vi "PID.vi"(0 "Refnum in":refnum<k21>, 1 "PID On/Off":bool, 2 "VISA resource name":refnum<visa-resource-name>, 3 "error in (no error)":errorcluster, 4 "Parameters":cluster{"P":dbl, "I":dbl, "D":dbl}, 5 "Plus Resistance":dbl, 6 "Goal Temperature (K)":dbl, 7 "Temperature":dbl) -> (8 "PID signal":dbl format="%.2f", 10 "error out":errorcluster)   [LabVIEW 2017]
uses:
  <vilib>/DAQmx/read.llb/DAQmx Read (Analog 1D DBL NChan 1Samp).vi
  <vilib>/DAQmx/miscellaneous.llb/DAQmx Fill In Error Info.vi
  <vilib>/addons/control/pid/pid.llb/PID (DBL).vi
  <vilib>/addons/control/pid/NI_PID_pid.lvlib
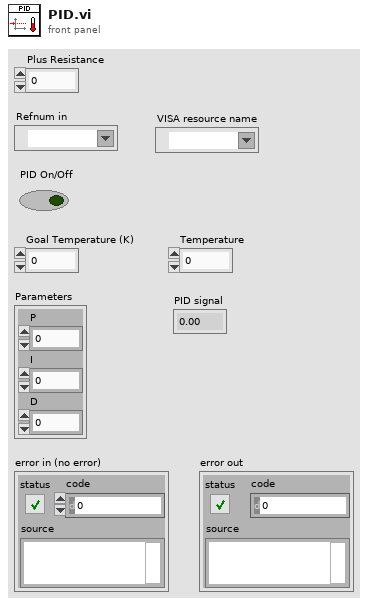
[diagram p1: front panel]
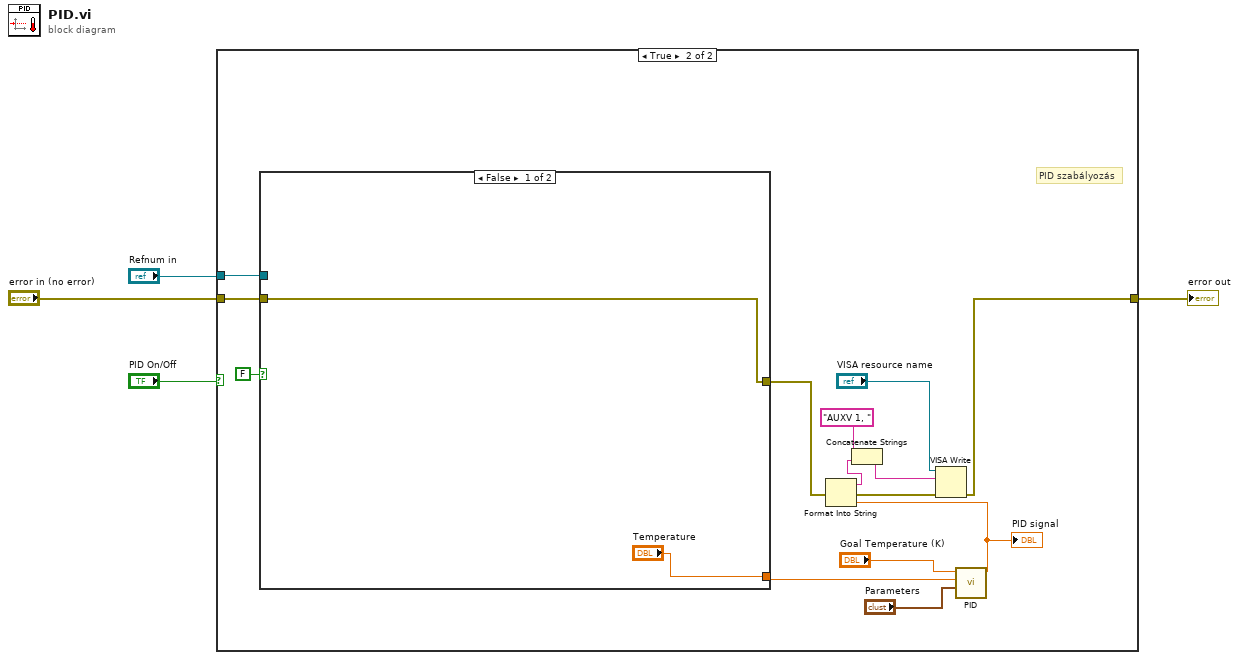
[diagram p0: block diagram]
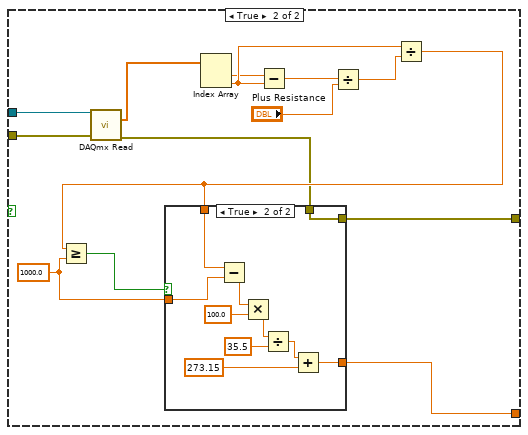
[diagram p3: hidden frame]
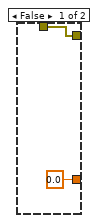
[diagram p4: hidden frame]
diagram:
  n1 = case shown="True" "PID On/Off" {
    tunnel: "error in (no error)" -> [w5 w18]
    tunnel: [w5 w14] -> w3
    tunnel: "Refnum in" -> [_ w19]
    frame False {
    }
    frame True {
      # "PID szabályozás"
      n2 = case shown="False" FALSE {
        tunnel: w19 -> [_ w27]
        tunnel: w18 -> [w20 w26]
        tunnel: ["Temperature" w24] -> w15
        tunnel: [w20 w22] -> w9
        frame False {
        }
        frame True {
          w34 = 1000.0 ("y")
          n3 = call-poly <vilib>:"DAQmx Read.vi"("task/channels in"=w27, "error in"=w26) -> ("data"=w31:dbl[], "error out"=w23:errorcluster)  [unwired: 11 in, 1 out]
          n4 = Index Array(array=w31) -> (element #1=w32:dbl, element #2=w33:dbl)  [unwired: 2 in]
          n5 = Subtract(x=w32, y=w33) -> (x-y=w28:dbl)
          n6 = Divide(x=w28, y="Plus Resistance") -> (x/y=w29:dbl)
          n7 = Divide(x=w33, y=w29) -> (x/y=w25:dbl)
          n8 = Greater Or Equal?(x=w25, y=w34) -> (x >= y?=w35:bool)
          n9 = case shown="True" w35 {
            tunnel: w34 -> [_ w43]
            tunnel: w25 -> [_ w42]
            tunnel: w23 -> [w37 w41]
            tunnel: [w37 w41] -> w22
            tunnel: [0.0 w38] -> w24
            frame False {
            }
            frame True {
              n10 = Subtract(x=w42, y=w43) -> (x-y=w45:dbl)
              n11 = Multiply(x=w45, y=100.0) -> (x*y=w47:dbl)
              n12 = Divide(x=w47, y=35.5) -> (x/y=w40:dbl)
              n13 = Add(x=w40, y=273.15) -> (x+y=w38:dbl)
            }
          }
        }
      }
      n14 = call-poly <vilib>:"PID.vi"("PID gains"="Parameters", "process variable"=w15, "setpoint"="Goal Temperature (K)") -> ("output"=w11:dbl)  [unwired: 7 in, 1 out]
      "PID signal" <- w11
      n15 = Format Into String(error in=w9, w11) -> (resulting string=w12:string, error out=w10:errorcluster)  [unwired: 2 in]
      n16 = Concatenate Strings("AUXV 1, " ("string"), w12) -> (w8:string)
      n17 = VISA Write(VISA resource name="VISA resource name", write buffer=w8, error in (no error)=w10) -> (error out=w14:errorcluster)  [unwired: 2 out]
    }
  }
  "error out" <- w3
